vi "Export Property.vi"(8 "error in (no error)":errorcluster, 9 "Value":string, 10 "Name":string, 11 "Node in":refnum<k20>) -> (0 "error out":errorcluster, 3 "Node out":refnum<k20>)   [LabVIEW 2013, in "JUnit for Azure Pipelines.lvclass"]
uses:
  JUnit for Azure Pipelines.lvclass
  <vilib>/xml/Close Reference(Node).vi
  <vilib>/xml/NI_XML.lvlib
  XML/XML.lvlib
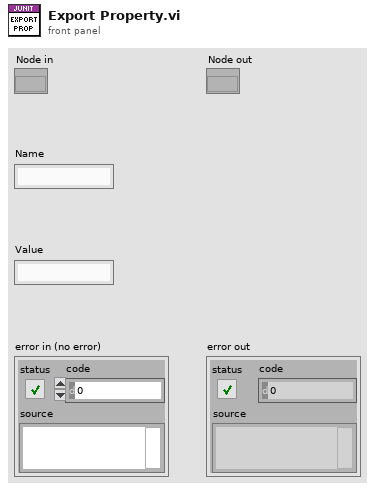
[diagram p1: front panel]
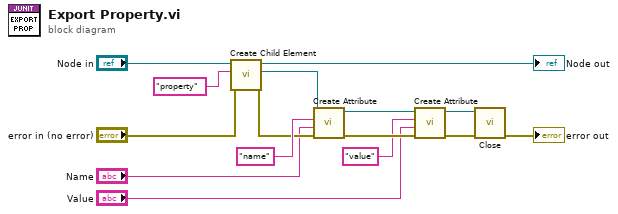
[diagram p0: block diagram]
diagram:
  n1 = call "Create Child Element.vi"("error in (no error)"="error in (no error)", "Name"="property" ("Tag Name"), "Element in"="Node in") -> ("error out"=w5:errorcluster, "Child Element"=w6:refnum<k20>, "Element out"=→"Node out":refnum<k20>)  [unwired: 6 in]
  n2 = call "Create Attribute.vi"("error in (no error)"=w5, "Value"="Name", "Name"="name" ("Attribute Name"), "Element in"=w6) -> ("error out"=w8:errorcluster, "Element out"=w9:refnum<k20>)  [unwired: 6 in]
  n3 = call "Create Attribute.vi"("error in (no error)"=w8, "Value"="Value", "Name"="value" ("Attribute Name"), "Element in"=w9) -> ("error out"=w3:errorcluster, "Element out"=w4:refnum<k20>)  [unwired: 6 in]
  n4 = call-poly <vilib>:"Close.vi"("error in (no error)"=w3, "node"=w4) -> ("error out"=→"error out":errorcluster)  [unwired: 7 in]
